vi "NullArray.vi"   [LabVIEW 2009]
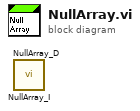
[diagram p0: block diagram]
diagram:
  n1 = call "NullArray_I.vi"() -> ()  [unwired: 11 in, 1 out]
  n2 = call "NullArray_D.vi"() -> ()  [unwired: 11 in, 1 out]
